vi "main.vi"() -> ()   [LabVIEW 2010]
panel:
  out "clock-wise\n sorted array":i32[][](array[numeric])
  out "left to right sorted array":i32[][](array[numeric])
  out "right to left\n sorted array":i32[][](array[numeric])
  out "NOIs from bottom\n half of image":dbl[][](array[numeric])
  out "NOIs from top\n half of image":dbl[][](array[numeric])
  out "Sorted points":cluster{"Y":dbl[], "Y":dbl[]}[](graph)
  out "Selected Points":cluster{"Y":dbl[], "Y":dbl[]}[](graph)
  in  "Array of NOI \n(Neurons of intetrest)\n coordinates":i32[][](array[numeric])
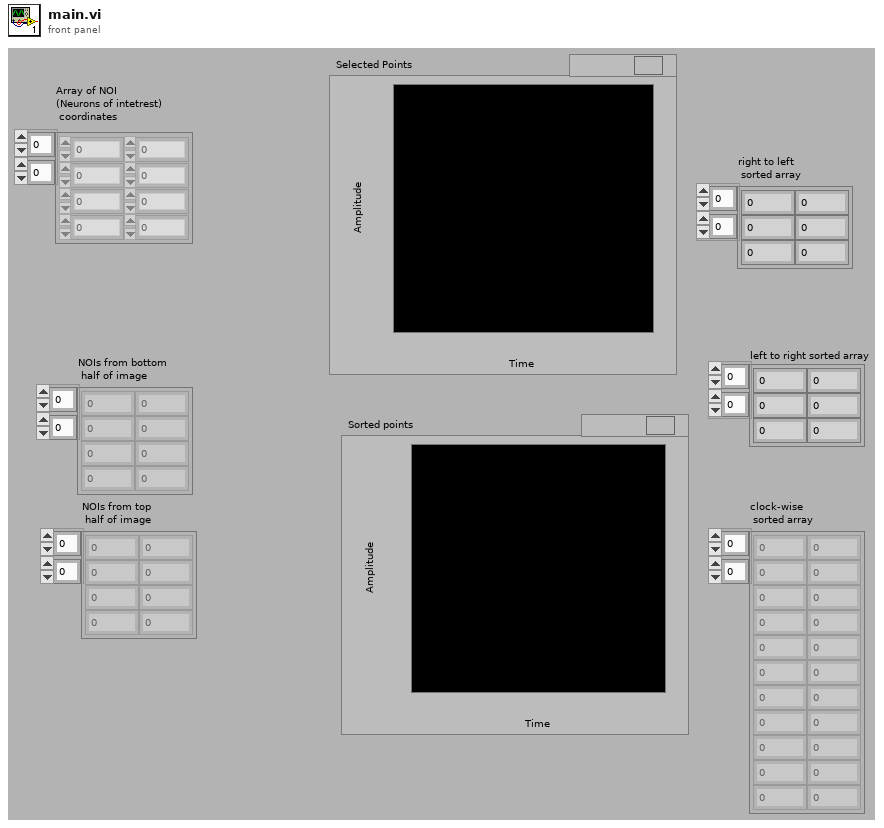
[diagram p1: front panel]
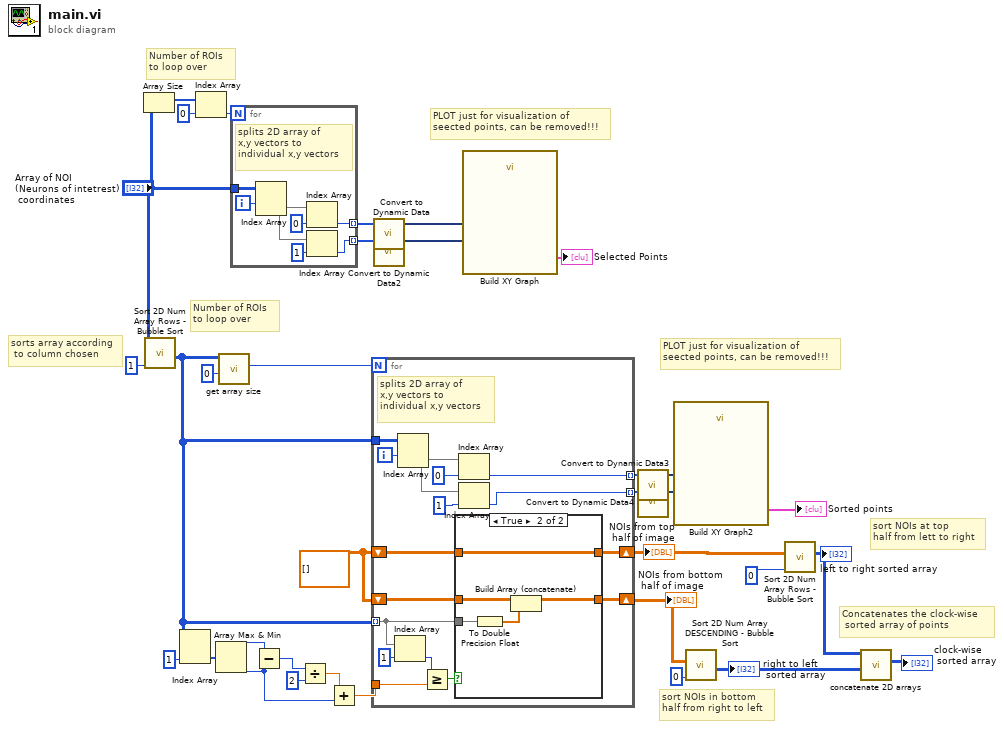
[diagram p0: block diagram]
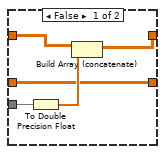
[diagram p2: hidden frame]
diagram:
  w15 = dbl[][] [] ("array")
  # "Concatenates the clock-wise\n sorted array of points"
  # "PLOT just for visualization of \nseected points, can be removed!!!"
  # "PLOT just for visualization of \nseected points, can be removed!!!"
  # "sort NOIs at top\nhalf from lett to right"
  # "sort NOIs in bottom\nhalf from right to left"
  # "sorts array according\n to column chosen"
  # "Number of ROIs\nto loop over"
  # "Number of ROIs\nto loop over"
  n1 = Array Size(array="Array of NOI \n(Neurons of intetrest)\n coordinates") -> (size(s)=w33:i32[])
  n2 = call "Sort 2D Num Array Rows - Bubble Sort.vi"("Column to Sort By"=1, "Input 2D Array"="Array of NOI \n(Neurons of intetrest)\n coordinates") -> ("Sorted Array"=w6:i32[][])  [unwired: 9 in]
  n3 = Index Array(array=w6, index (col)=1 ("disabled index (col)")) -> (element=w18:i32[])  [unwired: 1 in]
  n4 = Index Array(array=w33, index=0) -> (element=w32:i32)
  n5 = Array Max & Min(array=w18) -> (max value=w17:i32, min value=w11:i32)  [unwired: 2 out]
  n6 = call "get array size.vi"("index"=0, "array"=w6) -> ("array dimension"=w4:i32)  [unwired: 8 in]
  n7 = for {
    N: w32 -> [_]
    tunnel: "Array of NOI \n(Neurons of intetrest)\n coordinates" -> [w41]
    tunnel: [w36] -> w31 mode=indexing
    tunnel: [w35] -> w29 mode=indexing
    i -> [w40]
    # "splits 2D array of \nx,y vectors to\nindividual x,y vectors"
    n8 = Index Array(array=w41, index (row)=w40) -> (element=w37:i32[])  [unwired: 1 in]
    n9 = Index Array(array=w37, index=0) -> (element=w36:i32)
    n10 = Index Array(array=w37, index=1) -> (element=w35:i32)
  }
  n11 = Subtract(x=w17, y=w11) -> (x-y=w14:i32)
  n12 = Divide(x=w14, y=2) -> (x/y=w12:dbl)
  n13 = Add(x=w12, y=w11) -> (x+y=w16:dbl)
  n14 = for {
    N: w4 -> [_]
    tunnel: w6 -> [w57]
    tunnel: [w53] -> w21 mode=indexing
    tunnel: [w52] -> w20 mode=indexing
    tunnel: w6 -> [w47] mode=indexing
    tunnel: w16 -> [w49]
    shift-right: [w45] -> w9
    shift-left: w15 -> [w46]
    shift-right: [w44] -> w8
    shift-left: w15 -> [w43]
    i -> [w48]
    # "splits 2D array of \nx,y vectors to\nindividual x,y vectors"
    n15 = Index Array(array=w47, index=1) -> (element=w50:i32)
    n16 = Index Array(array=w57, index (row)=w48) -> (element=w54:i32[])  [unwired: 1 in]
    n17 = Greater Or Equal?(x=w50, y=w49) -> (x >= y?=w42:bool)
    n18 = case shown="True" w42 {
      tunnel: w47 -> [w60 w67]
      tunnel: w46 -> [w61 w63]
      tunnel: [w62 w63] -> w45
      tunnel: [w58 w65] -> w44
      tunnel: w43 -> [w58 w64]
      frame False {
        n19 = To Double Precision Float(number=w60) -> (double precision float=w59:dbl[])
        n20 = Build Array (concatenate)(w61, w59) -> (w62:dbl[][])
      }
      frame True {
        n21 = To Double Precision Float(number=w67) -> (double precision float=w66:dbl[])
        n22 = Build Array (concatenate)(w64, w66) -> (w65:dbl[][])
      }
    }
    n23 = Index Array(array=w54, index=0) -> (element=w53:i32)
    n24 = Index Array(array=w54, index=1) -> (element=w52:i32)
  }
  "NOIs from top\n half of image" <- w9
  "NOIs from bottom\n half of image" <- w8
  n25 = call "Convert to Dynamic Data"("Array"=w31) -> ("Dynamic Data Type"=w30:dynamicdata)  [unwired: 3 in]
  n26 = call "Convert to Dynamic Data2"("Array"=w29) -> ("Dynamic Data Type"=w28:dynamicdata)  [unwired: 3 in]
  n27 = call "Build XY Graph"("Y Input"=w28, "X Input"=w30) -> ("XY Graph"=→"Selected Points":cluster{"Y":dbl[], "Y":dbl[]}[])  [unwired: 3 in, 6 out]
  n28 = call "Convert to Dynamic Data3"("Array"=w21) -> ("Dynamic Data Type"=w22:dynamicdata)  [unwired: 3 in]
  n29 = call "Convert to Dynamic Data4"("Array"=w20) -> ("Dynamic Data Type"=w23:dynamicdata)  [unwired: 3 in]
  n30 = call "Build XY Graph2"("Y Input"=w23, "X Input"=w22) -> ("XY Graph"=→"Sorted points":cluster{"Y":dbl[], "Y":dbl[]}[])  [unwired: 3 in, 6 out]
  n31 = call "Sort 2D Num Array DESCENDING - Bubble Sort.vi"("Column to Sort By"=0, "Input 2D Array"=w8) -> ("Sorted Array"=w2:i32[][])  [unwired: 9 in]
  "right to left\n sorted array" <- w2
  n32 = call "Sort 2D Num Array Rows - Bubble Sort.vi"("Column to Sort By"=0, "Input 2D Array"=w9) -> ("Sorted Array"=w3:i32[][])  [unwired: 9 in]
  "left to right sorted array" <- w3
  n33 = call "concatenate 2D arrays.vi"("array 2"=w2, "array 1"=w3) -> ("concatenated array"=→"clock-wise\n sorted array":i32[][])  [unwired: 9 in]
